vi "Constants_global.vi"() -> ()   [LabVIEW 2012]
panel:
  in  "Public Folder":path=path "\\\\131.227.181.100\\Public"
  in  "EnFlo_Data_Central_Repository":path=path "/EnFlo_Data"
  in  "Data Folder Local":path=path "Please Run EnFlo Hub.vi"
  in  "Data Folder":path=path "Please Run EnFlo Hub.vi"
  in  "EnFlo SW Folder":path=path "Please Run EnFlo Hub.vi"
  in  "Traverse folder":path=path "Please Run EnFlo Hub.vi"
  in  "Run VI Folder":path=path "Please Run EnFlo Hub.vi"
  in  "All_Users":path=path "Please Run EnFlo Hub.vi"
  in  "Serial setups folder":path=path "Please Run EnFlo Hub.vi"
  in  "ADAM setups folder":path=path "Please Run EnFlo Hub.vi"
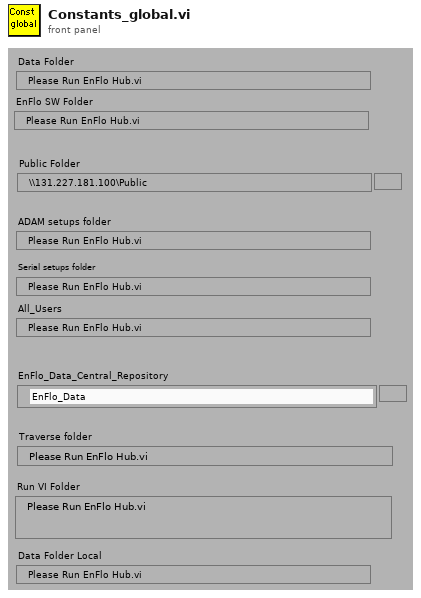
[diagram p1: front panel]
diagram:
